vi "Create Persistant Graph FRC1712.vi"(11 "XY":cluster{"x":dbl, "y":dbl}) -> (3 "Graph Plot":cluster{dbl[], dbl[]})   [LabVIEW 2019]
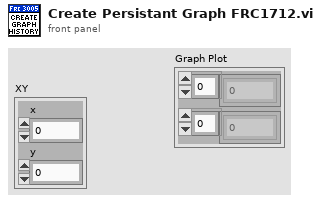
[diagram p1: front panel]
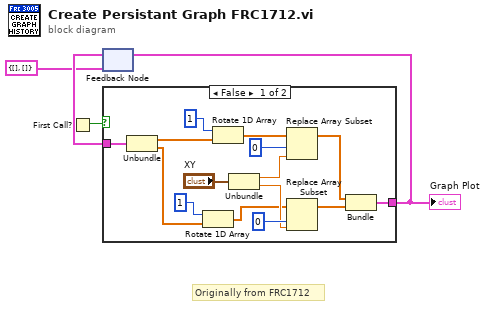
[diagram p0: block diagram]
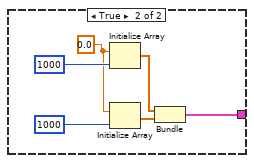
[diagram p2: hidden frame]
diagram:
  # "Originally from FRC1712"
  n1 = First Call?() -> (First Call?: T/F=w2:bool)
  n2 = feedback #1(cluster{dbl[], dbl[]} {[], []} ("output cluster")) -> (w3:cluster{dbl[], dbl[]})
  n3 = case shown="False" w2 {
    tunnel: [w9 w20] -> w4
    tunnel: w3 -> [w17 _]
    frame False {
      n4 = Unbundle(w17) -> (w16:dbl[], w6:dbl[])
      n5 = Rotate 1D Array(1:w6, 2:1 ("n")) -> (0:w5:dbl[])
      n6 = Rotate 1D Array(1:w16, 2:1 ("n")) -> (0:w15:dbl[])
      n7 = Unbundle("XY") -> ("x"=w13:dbl, "y"=w8:dbl)
      n8 = Replace Array Subset(array=w15, new element=w13, index=0) -> (w10:dbl[])
      n9 = Replace Array Subset(array=w5, new element=w8, index=0) -> (w11:dbl[])
      n10 = Bundle(w10, w11) -> (w9:cluster{dbl[], dbl[]})  [unwired: 1 in]
    }
    frame True {
      w23 = 0.0
      n11 = Initialize Array(w23, 1000 ("dimension size")) -> (w21:dbl[])
      n12 = Initialize Array(w23, 1000 ("dimension size")) -> (w22:dbl[])
      n13 = Bundle(w21, w22) -> (w20:cluster{dbl[], dbl[]})  [unwired: 1 in]
    }
  }
  "Graph Plot" <- w4
  n14 = feedback-in #1(w4) -> ()
